vi "Test MQTT-3.3.2-1.vi"(8 "error in (no error)":errorcluster) -> (0 "error out":errorcluster)   [LabVIEW 2013]
uses:
  source/Control Packets/ControlPacket/ControlPacket.lvclass/ControlPacket.ctl
  <vilib>/addons/_JKI Toolkits/Caraya/classes/Test/Test.lvclass
  <vilib>/addons/_JKI Toolkits/Caraya/classes/Assert/Assert.lvclass
  source/Control Packets/PUBLISH/PUBLISH.lvclass
  source/Control Packets/ControlPacket/ControlPacket.lvclass
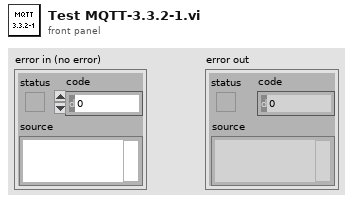
[diagram p1: front panel]
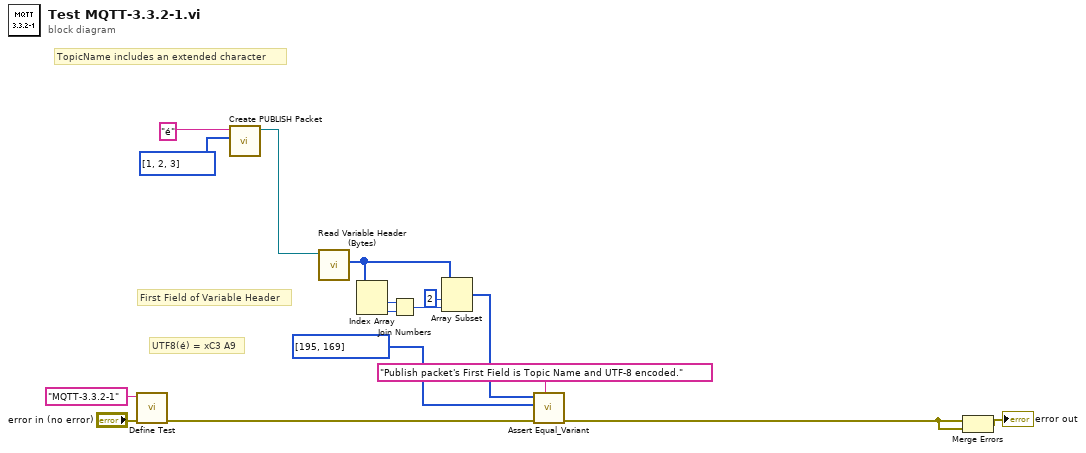
[diagram p0: block diagram]
diagram:
  # "First Field of Variable Header"
  # "UTF8(é) = xC3 A9"
  # "TopicName includes an extended character"
  n1 = call <vilib>:"Define Test.vi"("error in (no error)"="error in (no error)", "Label (VI Title)"="MQTT-3.3.2-1") -> ("error out"=w13:errorcluster)  [unwired: 9 in]
  n2 = call "Create PUBLISH Packet.vi"("Payload"=u8[] [1, 2, 3], "Topic Name"="é" ("Client ID (empty: generate new)")) -> ("PUBLISH"=w3:refnum<class "PUBLISH.lvclass">)  [unwired: 7 in, 2 out]
  n3 = call "Read Variable Header (Bytes).vi"("ControlPacket in"=w3) -> ("Variable Header (Bytes)"=w6:u8[])  [unwired: 9 in, 1 out]
  n4 = Index Array(array=w6) -> (element #1=w7:u8, element #2=w8:u8)  [unwired: 2 in]
  n5 = Join Numbers(hi=w7, lo=w8) -> ((hi.lo)=w4:u16)
  n6 = Array Subset(array=w6, index=2, length=w4) -> (w2:u8[])
  n7 = call <vilib>:"Assert Equal_Variant.vi"("Label"="Publish packet's First Field is Topic Name and UTF-8 encoded.", "error in (no error)"=w13, "Y"=u8[] [195, 169] ("subarray"), "X"=w2) -> ("error out"=w10:errorcluster)  [unwired: 7 in]
  n8 = Merge Errors(w10, w10) -> (→"error out":errorcluster)
